vi "test_Configure Response_DataChannels Hierarchy Error.vi"(8 "error in (no error)":errorcluster, 11 "TestCase in":refnum<class "Instrument Addon Scripting API Messages Unit Tests.lvclass">) -> (0 "error out":errorcluster, 3 "TestCase out":refnum<class "Instrument Addon Scripting API Messages Unit Tests.lvclass">)   [LabVIEW 2018, in "Instrument Addon Scripting API Messages Unit Tests.lvclass"]
uses:
  Instrument Addon Scripting API Messages Unit Tests.lvclass
  APIs/Scripting API/TypeDefs/Wait Response Settings.ctl
  APIs/Scripting API/TypeDefs/Linked Channel.ctl
  <vilib>/NI Veristand/Custom Device API/Custom Device Item Ref.ctl
  Instrument Addon Scripting API Messages Unit Tests.lvclass/Instrument Addon Scripting API Messages Unit Tests.ctl
  Addon/Addon Shared/SubVIs/Constants.vi
  <vilib>/NI/NI VeriStand Advanced SysDef API/_SubVIs/SysDef.Search.GUID.vi
  APIs/Scripting API/Messages/Configure Response - Wait (sec).vi
  <vilib>/addons/_JKI Toolkits/VI Tester/TestCase.llb/TestCase.lvclass
  Instrument Addon Scripting API Test Assets/Instrument Addon Scripting API Test Assets.lvclass
  APIs/Scripting API/Instrument Addon Scripting API.lvlib
  <vilib>/NI Veristand/Custom Device API/Custom Device API.lvlib
  <vilib>/NI/NI VeriStand Advanced SysDef API/SysDef API/Advanced System Definition.lvlib
  Addon/Addon Shared/Instrument Addon Shared.lvlib
  C:/Program Files (x86)/National Instruments/LabVIEW 2018/vi.lib/addons/_JKI Toolkits/VI Tester/TestCase.llb/TestCase.lvclass
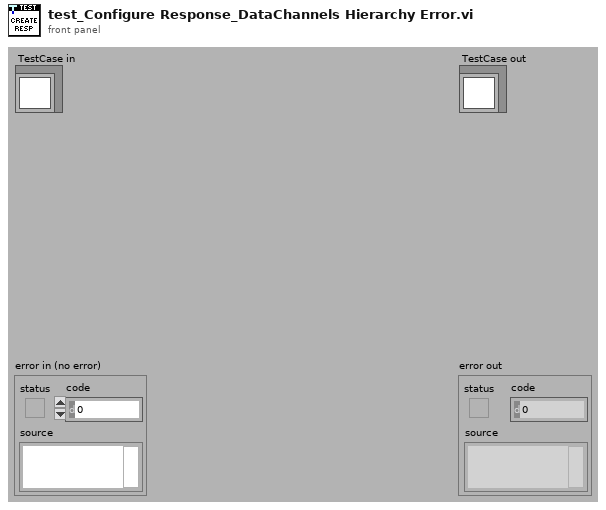
[diagram p1: front panel]
types:
  T1 = typedef "Instrument Addon Scripting API.lvlib/Wait Response Settings.ctl" = cluster{"Response Format":string, "Linked Channels":T2[], "Wait value (sec)":dbl, "Use Wait Channel":bool, "Channel Refnum":T3}
  T2 = typedef "Instrument Addon Scripting API.lvlib/Linked Channel.ctl" = cluster{"Variable Name":string, "Channel Refnum":T3}
  T3 = typedef "Custom Device API.lvlib/Custom Device Item Ref.ctl" = u64
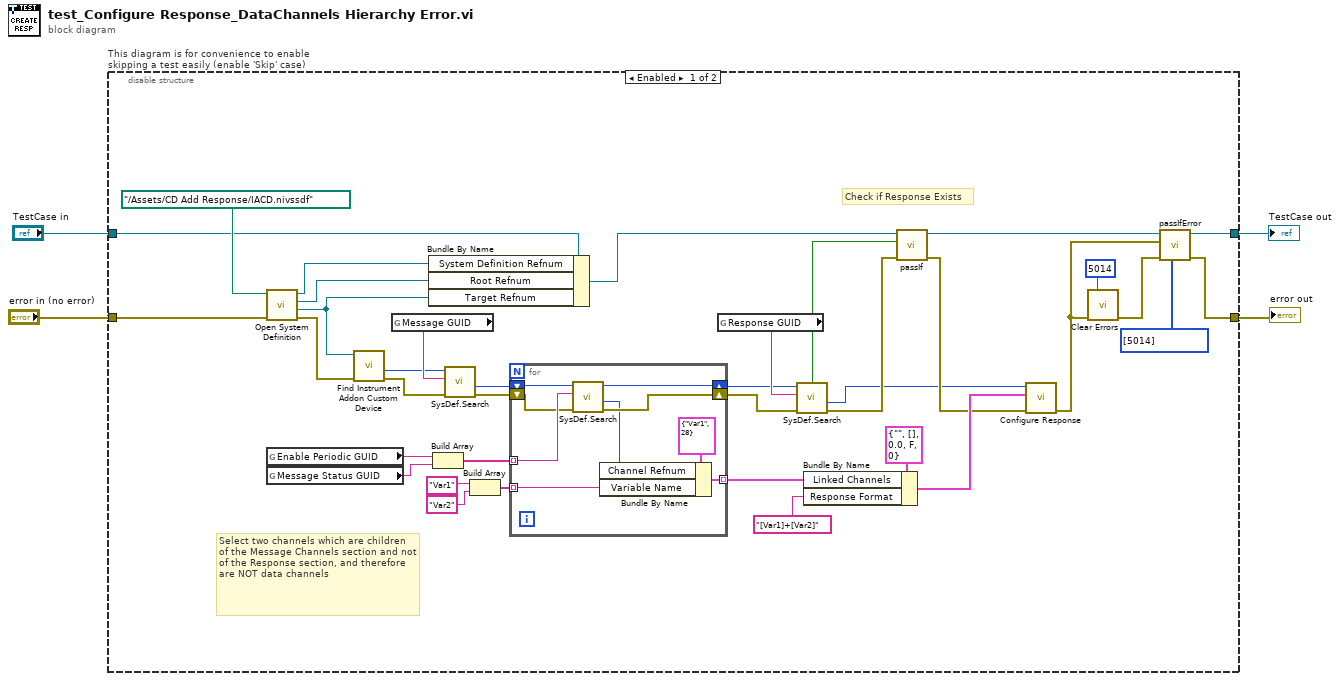
[diagram p0: block diagram]
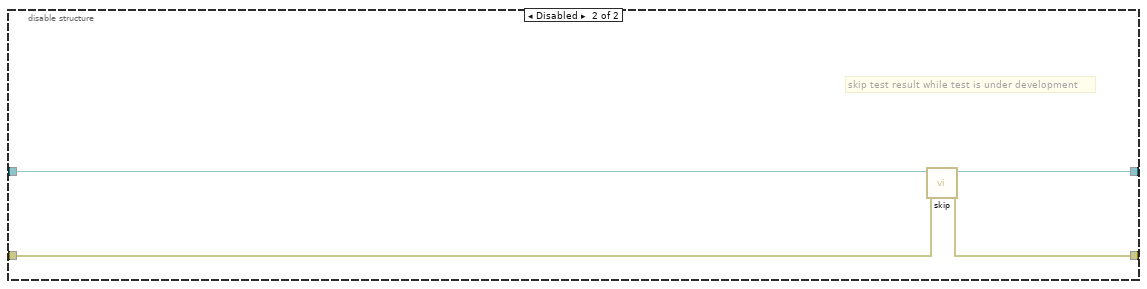
[diagram p2: hidden frame]
diagram:
  n1 = disable-structure "This diagram is for convenience to enable skipping a test easily (enable 'Skip' case)" shown="Enabled" {
    disable-tunnel: "TestCase in" -> [w12 w54]
    disable-tunnel: [w31 w52] -> w1
    disable-tunnel: [w30 w53] -> w3
    disable-tunnel: "error in (no error)" -> [w40 w51]
    frame Enabled {
      # "Select two channels which are children of the Message Channels section and not of the Response section, and therefore are NOT data channels"
      # "Check if Response Exists"
      n2 = call "Open System Definition.vi"("error in (no error)"=w40, "System Definition File"=path "../Assets/CD Add Response/IACD.nivssdf" ("SDF file")) -> ("error out"=w39:errorcluster, "Target Refnum"=w10:refnum<k24>, "Root Refnum"=w9:refnum<k24>, "System Definition Refnum"=w8:refnum<k24>)  [unwired: 6 in]
      n3 = global read "Constants.vi" "Enable Periodic GUID"() -> (w23:string)
      n4 = global read "Constants.vi" "Message Status GUID"() -> (w22:string)
      n5 = call "Find Instrument Addon Custom Device.vi"("error in"=w39, "target in"=w10) -> ("error out"=w26:errorcluster, "NodeID"=w25:u64)  [unwired: 7 in, 1 out]
      n6 = global read "Constants.vi" "Message GUID"() -> (w27:string)
      n7 = Bundle By Name(cluster=w12, "System Definition Refnum"=w8, "Root Refnum"=w9, "Target Refnum"=w10) -> (w11:refnum<class "Instrument Addon Scripting API Messages Unit Tests.lvclass">)
      n8 = Build Array(w23, w22) -> (w21:string[])
      n9 = call-poly <vilib>:"SysDef.Search.vi"("error in (no error)"=w26, "GUID"=w27, "nodeID"=w25) -> ("error out"=w19:errorcluster, "Value out"=w20:u64)  [unwired: 5 in, 2 out]
      n10 = Build Array("Var1" ("Response Format"), "Var2" ("Response Format")) -> (w14:string[])
      n11 = for {
        tunnel: w21 -> [w49] mode=indexing
        shift-right: [w46] -> w18
        shift-left: w20 -> [w50]
        shift-right: [w47] -> w17
        shift-left: w19 -> [w48]
        tunnel: w14 -> [w44] mode=indexing
        tunnel: [w42] -> w13 mode=indexing
        n12 = call-poly <vilib>:"SysDef.Search.vi"("error in (no error)"=w48, "GUID"=w49, "nodeID"=w50) -> ("error out"=w47:errorcluster, "Value out"=w43:u64, "nodeID out"=w46:u64)  [unwired: 5 in, 1 out]
        n13 = Bundle By Name(cluster=T2 {"Variable Name"="Var1", "Channel Refnum"=28} ("Linked Channel"), "Channel Refnum"=w43, "Variable Name"=w44) -> (w42:T2)
      }
      n14 = global read "Constants.vi" "Response GUID"() -> (w37:string)
      n15 = call-poly <vilib>:"SysDef.Search.vi"("error in (no error)"=w17, "GUID"=w37, "nodeID"=w18) -> ("error out"=w24:errorcluster, "Value out"=w5:u64, "Found?"=w36:bool)  [unwired: 5 in, 1 out]
      n16 = Bundle By Name(cluster=T1 {"Response Format"="", "Linked Channels"=[], "Wait value (sec)"=0.0, "Use Wait Channel"=FALSE, "Channel Refnum"=0} ("Settings"), "Linked Channels"=w13, "Response Format"="[Var1]+[Var2]") -> (w34:T1)
      n17 = call-dynamic "passIf.vi"("error in (no error)"=w24, "pass"=w36, "TestCase in"=w11) -> ("error out"=w33:errorcluster, "TestCase out"=w32:refnum<class "Instrument Addon Scripting API Messages Unit Tests.lvclass">)  [unwired: 7 in]
      n18 = call-poly "Configure Response.vi"("error in (no error)"=w33, "settings"=w34, "reponse refnum in"=w5) -> ("error out"=w7:errorcluster)  [unwired: 7 in, 1 out]
      n19 = call <vilib>:"Clear Errors.vi"("error in (no error)"=w7, "specific error code to clear (0: all)"=5014) -> ("error out"=w28:errorcluster)  [unwired: 4 in, 1 out]
      n20 = call-dynamic "passIfError.vi"("passing error codes (default = any error code)"=i32[] [5014], "error in (no error)"=w28, "error"=w7, "TestCase in"=w32) -> ("error out"=w30:errorcluster, "TestCase out"=w31:refnum<class "Instrument Addon Scripting API Messages Unit Tests.lvclass">)  [unwired: 6 in]
    }
    frame Disabled {
      # "skip test result while test is under development"
      n21 = call <vilib>:"skip.vi"("error in (no error)"=w51, "TestCase in"=w54) -> ("error out"=w53:errorcluster, "TestCase out"=w52:refnum<class "Instrument Addon Scripting API Messages Unit Tests.lvclass">)  [unwired: 8 in]
    }
  }
  "error out" <- w3
  "TestCase out" <- w1
